vi "ProtocolAnalysis 3.vi"(8 "error in":errorcluster caption="错误输入", 11 "IP":refnum<k5>) -> (0 "error out":errorcluster caption="错误输出", 1 "Disconnected":bool, 3 "IP 2":refnum<k5>)   [LabVIEW 2015]
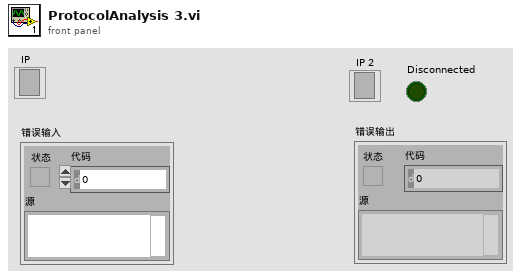
[diagram p1: front panel]
types:
  T1 = enum16{"Standard", "Buffered", "CRLF", "Immediate"}
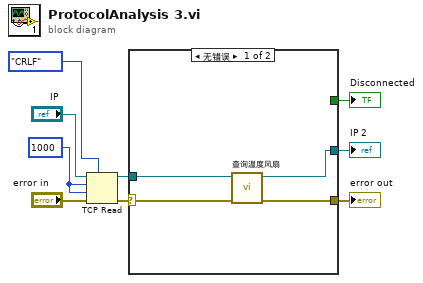
[diagram p0: block diagram]
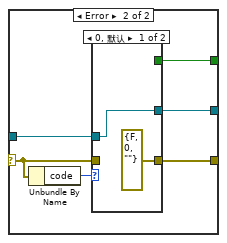
[diagram p2: hidden frame]
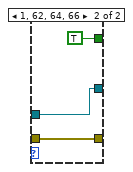
[diagram p3: hidden frame]
diagram:
  w2 = 1000 ("timeout ms (25000)")
  n1 = TCP Read(connection ID="IP", bytes to read=w2, error in (no error)="error in", 7:T1."CRLF" ("mode (standard)"), 9:w2) -> (connection ID out=w4:refnum<k5>, error out=w3:errorcluster)  [unwired: 1 out]
  n2 = case shown="无错误" w3 {
    selector: w3 -> [w11 w18]
    tunnel: [w10 w17] -> w5
    tunnel: w4 -> [w13 w16]
    tunnel: [w12 w15] -> w8
    tunnel: [_ w14] -> w7
    frame No Error {
      n3 = call "查询温度风扇.vi"("error in (no error)"=w11, "TCP Network Connection in"=w13) -> ("error out"=w10:errorcluster, "TCP Network Connection out"=w12:refnum<k5>)  [unwired: 8 in]
    }
    frame Error {
      n4 = Unbundle By Name(w18) -> ("code"=w19:i32)
      n5 = case shown="0, 默认" w19 {
        tunnel: w18 -> [_ w22]
        tunnel: [errorcluster {"status"=FALSE, "code"=0, "source"=""} ("error IO") w22] -> w17
        tunnel: w16 -> [w21 w23]
        tunnel: [w21 w23] -> w15
        tunnel: [_ TRUE] -> w14
        frame 0, Default {
        }
        frame 1, 62, 64, 66 {
        }
      }
    }
  }
  "error out" <- w5
  "IP 2" <- w8
  "Disconnected" <- w7
